vi "_Fade Out(String).vi"(6 "Fade (Exponential)":T1, 8 "error in":errorcluster, 10 "Fade time (ms)":string, 11 "VI Reference (calling VI)":refnum<vi>) -> (0 "error out":errorcluster, 3 "dup VI Reference":refnum<vi>)   [LabVIEW 2012]
doc: "Produces a \"Fade Out\" on the VI from which a reference has been provided.\n\nThe string input for Fade time allows the use of string-based arguments without the need to convert to a number."
uses:
  _fadetype.ctl
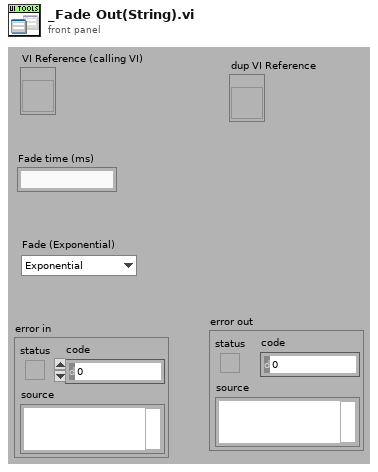
[diagram p1: front panel]
types:
  T1 = typedef "_fadetype.ctl" = enum16{"Exponential", "Linear"}
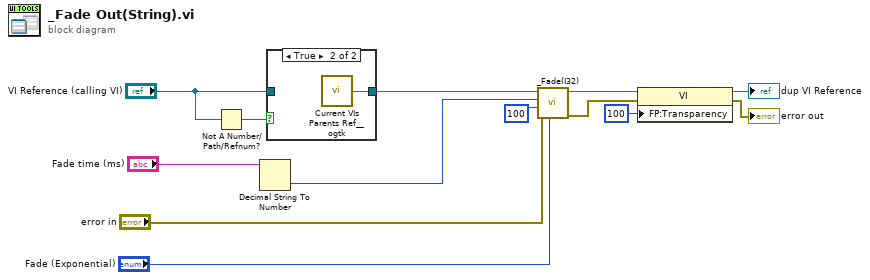
[diagram p0: block diagram]
diagram:
  n1 = Not A Number/Path/Refnum?(number/path/refnum="VI Reference (calling VI)") -> (NaN/Path/Refnum?=w13:bool)
  n2 = Decimal String To Number(string="Fade time (ms)") -> (number=w2:i32)  [unwired: 3 out]
  n3 = case shown="True" w13 {
    tunnel: "VI Reference (calling VI)" -> [w14 _]
    tunnel: [w14 w15] -> w3
    frame False {
    }
    frame True {
      n4 = call <userlib>:"Current VIs Parents Ref__ogtk.vi"() -> ("Calling VI's Reference"=w15:refnum<vi>)  [unwired: 2 out]
    }
  }
  n5 = call "_Fade(I32).vi"("Fade (Exponential)"="Fade (Exponential)", "error in"="error in", "Target Transparency (0)"=u8 100 ("Front Panel Window:Transparency"), "Fade time (ms)"=w2, "VI Reference (calling VI)"=w3) -> ("error out"=w7:errorcluster, "dup VI Reference"=w9:refnum<vi>)  [unwired: 5 out]
  n6 = property class="VI"(reference=w9, error in=w7, "FP:Transparency"=u8 100 ("Front Panel Window:Transparency")) -> (reference out=→"dup VI Reference":refnum<vi>, error out=→"error out":errorcluster)
